vi "Start Test.vi"(8 "error in (no error)":errorcluster, 11 "Model in":refnum<class "Model.lvclass">) -> (0 "error out":errorcluster, 3 "Model out":refnum<class "Model.lvclass">)   [LabVIEW 2016, in "Model.lvclass"]
uses:
  Model.lvclass
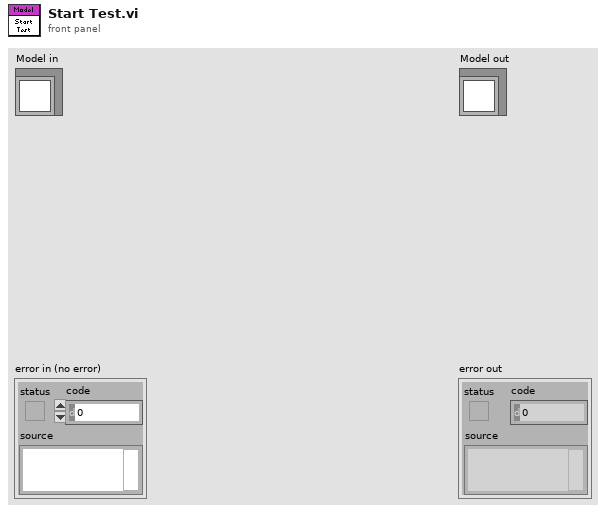
[diagram p1: front panel]
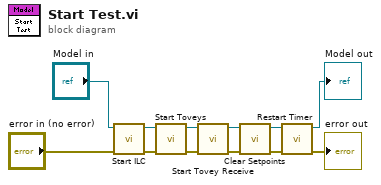
[diagram p0: block diagram]
diagram:
  n1 = call "Start ILC.vi"("error in (no error)"="error in (no error)", "Model in"="Model in") -> ("error out"=w10:errorcluster, "Model out"=w7:refnum<class "Model.lvclass">)  [unwired: 8 in]
  n2 = call "Start Toveys.vi"("error in (no error)"=w10, "Model in"=w7) -> ("error out"=w9:errorcluster, "Model out"=w6:refnum<class "Model.lvclass">)  [unwired: 8 in]
  n3 = call "Start Tovey Receive.vi"("error in (no error)"=w9, "Model in"=w6) -> ("error out"=w12:errorcluster, "Model out"=w5:refnum<class "Model.lvclass">)  [unwired: 8 in]
  n4 = call "Clear Setpoints.vi"("error in (no error)"=w12, "Model in"=w5) -> ("error out"=w11:errorcluster, "Model out"=w4:refnum<class "Model.lvclass">)  [unwired: 8 in]
  n5 = call "Restart Timer.vi"("error in (no error)"=w11, "Model in"=w4) -> ("error out"=→"error out":errorcluster, "Model out"=→"Model out":refnum<class "Model.lvclass">)  [unwired: 8 in]
